vi "AlliGator Plot Fit Parameter vs Intensity v2.vi"(6 "Fit Parameter":T1, 7 "Lifetime Graph refnum":refnum<vi>, 8 "error in (no error)":errorcluster, 9 "ROI idx (2147483647: all ROIs)":i32=-1, 11 "Data Value Reference in":refnum<data-value>) -> (0 "error out":errorcluster, 3 "Data Value Reference out":refnum<data-value>)   [LabVIEW 2021, in "AlliGator Decay Fit Parameter Map.lvlib"]
doc: "Creates scatter plot of selected parameter vs intensity for all ROIs and sends it to the <B>Lifetime & Other Parameters Graph</B>."
uses:
  AlliGator Decay Fit Parameter Map.lvlib
  AlliGator Internal Variables v2.ctl
  <vilib>/vision/Image Controls.llb/IMAQ Image.ctl
  AlliGator Gate Image Set.ctl
  AlliGator FLI Dataset Type.ctl
  AlliGator Data Series Type.ctl
  AlliGator Dataset Channel.ctl
  AlliGator Gate Arithmetic.ctl
  AlliGator Displayed Image.ctl
  Image/Named ROI Description.ctl
  AlliGator Decay Metadata v3.ctl
  AlliGator Decay Background Subtraction Info.ctl
  AlliGator Baseline Subtraction Method.ctl
  Graphs/XY Graph/XY Graph Plot Shift Parameters.ctl
  Graphs/XY Graph/XY Graph Plot Shift Method.ctl
  AlliGator Decay Extrapolation Parameters.ctl
  Phasor/Calibration Phasor (m, phi).ctl
  Phasor/Phasor Reference Series.ctl
  Phasor/Phasor Calibration Map v2.ctl
  Phasor/Phasor (g, s).ctl
  AlliGator Raw Phasor Plot Data v4.ctl
  Phasor/Phasor Standard Deviation Options.ctl
  AlliGator Phasor Multi-Harmonic Data.ctl
  Phasor/Phasor Harmonic Data.ctl
  AlliGator Decay Fit Options & Parameters v2.ctl
  Fits/IRF(X)PSED/Decay Fit Options v2.ctl
  Fits/Decay Convolution/Decay Model.ctl
  Fits/Residual Type.ctl
  Fits/IRF(X)PSED/Fit Weights Type.ctl
  Fits/Non-linear Fitting Method v2.ctl
  Fits/Fit Calculation Method.ctl
  Fits/Non-linear Fitting Algorithm.ctl
  AlliGator Decay Fit Parameter Constraints 2.ctl
  Fits/IRF(X)PSED/Decay Fit Parameters In List.ctl
  Fits/IRF(X)PSED/MLE Baseline Offset Type.ctl
  AlliGator Decay Preprocessing Parameters.ctl
  Fits/IRF(X)PSED/Decay Fit Parameters & Derived Quantities List.ctl
  AlliGator Variables List.ctl
  Graphs/LabVIEW Plot Interpolation.ctl
  Graphs/Plot Point Style.ctl
  Variant/Variant to Data/Variant to U16.vi
  AlliGator Files.lvlib
  Graphs/XY Graph/XY Graph Add-Ons.lvlib
  AlliGator Globals, Variables & Constants.lvlib
  Image/Image.lvlib
  Notebook/Notebook.lvlib
  Rich Text Box/Rich Text Box.lvlib
  Variant/Variant to Data/Variant to Data.lvlib
  <vilib>/vision/NI_Vision_Development_Module.lvlib
  Graphs/Graphs.lvlib
  Phasor/Phasor.lvlib
  AlliGator Decay Preprocessing.lvlib
  AlliGator Phasor Graph.lvlib
  AlliGator Phasor Plot.lvlib
  AlliGator Source Image.lvlib
  Fits/Fits.lvlib
  AlliGator Internal Variables.lvlib
  AlliGator Decay Fit.lvlib
  AlliGator Settings.lvlib
  AlliGator Dual-Channel Datasets.lvlib
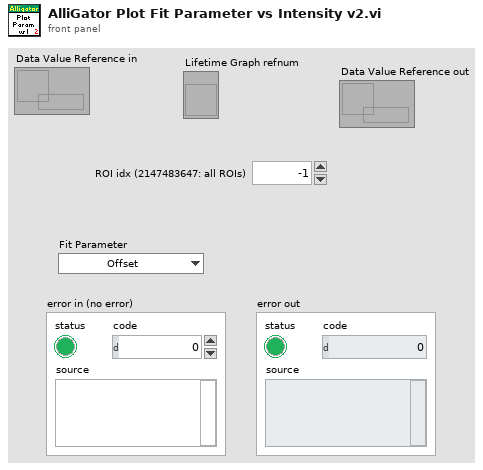
[diagram p1: front panel]
types:
  T1 = typedef "Fits.lvlib/Decay Fit Parameters & Derived Quantities List.ctl" = enum16{"Offset", "Baseline", "A_1", "tau_1", "A_2", "tau_2", "<tau>_a", "f1_a", "f2_a", "<tau>_i", "f1_i", "f2_i", "-", "R^2", "Chi^2"}
  T2 = typedef "AlliGator Globals, Variables & Constants.lvlib/AlliGator Variables List.ctl" = enum16{"---- GUI ----", "Initialization Status", "State Indicators Refnum", "Original AlliGator Menu Items", "Current Action Loop State", "Script in progress", "Playback", "Loop Playback", "Search ROI Used", "Search ROI", "Decay Graph Max Legend Size", "Intensity Graph Max Legend Size", "Decay Statistics Graph Max Legend Size", "Phasor Graph Max Legend Size", "Phasor Ratio Graph Max Legend Size", "Lifetime Graph Max Legend Size", "---- Files ----", "Export Dataset Frames as Individual Files", "Show Batch Export Help Balloons", "Frames in Dataset", "ptu File Frame Start Indices", "Current Frame in Dataset", "Current Frame Timestamp", "------ Python Plugins ------", "Python Plugins Information", "Python Session", "Valid Python Session?", "---- Source Image ----", "Dataset Loaded", "Dataset Metadata", "Dataset Channel", "Dataset Data Description", "Background Dataset Metadata", "Background Dataset Channel", "Background Dataset Data Description", "Background File Subtraction", "Background File Path", "Background File Pile-up Correction", "Background File Pixel Well Capacity", "Background File Scaling Factor", "Source Image ROIs", "Current Source Image ROI", "Source Image ROI Event Refnum", "X_Source Image Display Range", "X_Source Image Palette Information", "Source Image Palette List", "Source Image Scale", "Current Dataset Load Settings", "Source Image:ROI Overlay Color", "---- Image Profile Window ----", "Image Profile:Overlay ROI in Source Image", "Image Profile Window Event Refnum", "Image Profile:IntensityType", "Image Profile:Intensity Average Type", "Image Profile:Intensity-weighted SDV", "Image Profile:Box Profile Type", "Image Profile Window Open", "Image Profile:Plotted Fit Parameter", "X_Type of Displayed Image", "X_Time Gate Slider", "Dataset Path", "Source Image Overlay to Erase", "Is Displayed Image Accumulated", "White Light Image Modified", "Mask Image Modified", "Macrotime Gate Separation", "------ Phasor Graph -------", "Phasor Graph:Show Line", "---- Phasor Plot ---", "Phasor Plot Parameters Changed", "FLI Dataset Modified since last Phasor Plot Calculation", "Phasor Harmonics Data", "Selected Phasor Harmonics", "Phasor Harmonic Manager Event Refnum", "Phasor Plot ROIs", "Current Phasor Plot ROI", "Phasor Plot ROI Event Refnum", "Phasor Plot Image Reference Points", "Phasor Plot Computed", "Phasor Plot Palette Information", "Phasor Plot Palette List", "Phasor Ratio Palette Information", "Phasor Ratio Palette List", "Phasor Image Scale", "Phasor Plot Image Overlay to Erase", "Phasor Plot Image Elements to Update", "Current Phasor Plot Calculation Parameters", "Current Phasor Calibration Options", "Reset Cumulated Phasor Plot", "Phasor Ratio Reference 1", "Phasor Ratio Lifetime Reference 1", "Phasor Ratio Reference 1 Frequency", "Phasor Ratio Reference 2", "Phasor Ratio Lifetime Reference 2", "Phasor Ratio Reference 2 Frequency", "---- Decay Analysis ----", "Number of Selected Decays to Fit", "LS Fit Results", "LAR Fit Results", "BS Fit Results", "Last Decay Max - Min", "Best Fit Parameters", "Best Fit Parameter Names", "Actual Size X", "Actual Size Y", "Binning X", "Binning Y", "Actual # Gates", "Dataset Number", "Gates to...", "Gates Skipped", "Gates to keep", "Gate Step", "Gate Separation", "Reversed Gates", "Pile-up Correction", "Pixel Well Capacity", "Background Subtracted", "Background Subtraction Method", "Background Definition Range", "Background File (deprecated)", "Number of Dataset Accumulated", "Array of Accumulated Dataset Paths", "Do Averaged Datasets", "Destination File Path", "Process Plot Target", "Use 1/D as Phasor Frequency", "---- Decay Fit Parameter Map -----", "Decay Fit Parameter Map Palette Information", "Decay Fit Parameter Map Palette List", "Local Decay Graph Window Event Refnum", "------- Local Decay Window ---------", "Use normalized IRF for convolution", "----- Miscellaneous ----", "Skippable Dialog Windows Status"}
  T3 = typedef "Graphs.lvlib/Plot Point Style.ctl" = enum16{"not defined", "None", "Empty Circle", "Filled Circle", "Thick Circle", "Dotted Circle", "Empty Square", "Filled Square", "Thick Square", "Dotted Square", "Small Filled Square", "Dot", "Cross", "Tiny Cross", "Large X", "Small x", "Diamond", "Small Empty Square"}
  T4 = typedef "Image.lvlib/Named ROI Description.ctl" = cluster{"ROI Descriptor":T5, "ROI Name":string, "Overlay Color":u32}
  T5 = typedef "ROI Descriptor" = cluster{"Global Rectangle":i32[], "Contours":cluster{"ID":enum32{"External", "Internal"}, "Type":u32, "Coordinates":i32[]}[]}
  T6 = typedef "AlliGator Internal Variables.lvlib/AlliGator Internal Variables v2.ctl" = cluster{"Displayed Image":T7, "White Light Image":T7, "Mask Image":T7, "ROI Mask Image":T7, "Current Dataset Images 1":T8, "Background Dataset Images 1":T8, "Current Dataset Images 2":T8, "Background Dataset Images 2":T8, "Current Dataset Arithmetic Images":T8, "Accumulated Dataset Images 1":T8, "Accumulated Dataset Images 2":T8, "Accumulated Dataset Arithmetic Images":T8, "Phasor Plot Image":T7, "Decay Fit Parameter Map Image":T7, "Single Data Point Path":path, "White Light Image Path":path, "Mask Image Path":path, "Time-Series Folder":path, "[Time-Series Paths]":path[], "Current Dataset":i32, "Single Dataset Type":T9, "Current Folder":string, "AlliGator Data Series Type":T10, "# Datasets":i32, "Dual-Channel Dataset":bool, "Selected Channel Name":string, "Dataset Channel":T11, "Channel Arithmetic":T12, "Dual-Channel Background Dataset":bool, "Background Channel":T11, "Dual-Channel Accumulated Dataset":bool, "Start Time":dbl, "[Time-Series Timestamps]":dbl[], "[Intensity Corrections]":dbl[], "Time Series Script":bool, "Type of Displayed Image":T13, "Gate Image Slide":u16, "# Gates":i32, "ROIs":T4[], "ROI Decay":cluster{"t Array":dbl[], "I Array":dbl[]}, "Valid Decay":bool, "Decay  Metadata":T14, "Reference Decay Plot Name":string, "Reference Decay":cluster{"t Array":dbl[], "I Array":dbl[]}, "Decay Shift Plot":cluster{"Time Stamps":dbl[], "Decay Shifts":dbl[]}, "[Decays Max Values]":sgl[], "[Decays Min Values]":sgl[], "Calibration Phasor":T20, "Calibration Phasor Series":T21, "Phasor Calibration Map":T22, "Calibration Map MD5 Digest":string, "Last Raw Phasor":T23, "Last Calibrated Phasor":T23, "Last Calibrated Phasor SDV":T23, "Phasor Graph:Phasor Plot":cluster{"g Array":dbl[], "s Array":dbl[]}, "Phasor Graph:Phasor SDV Plot":cluster{"g Array":dbl[], "s Array":dbl[]}, "[Phasor Graph:Raw Phasor Plots]":T24[], "Phasor Plot locked to Ref 1":i32, "[Phasor Plot(s) locked to Ref 1]":i32[], "[Phasor Plot(s) locked to Ref 2]":i32[], "[Pixel Phasors]":T23[], "[[Sum Image]]":dbl[][], "[[CSG Phasors]]":csg[][], "[[Valid Pixel?]]":bool[][], "I/m/phi Dataset":cluster{"I/m/phi Dataset?":bool, "Base Frequency":dbl[unit], "Harmonic Orders":u8[]}, "Multi Phasor Plot Data":T26, "Decay Fit Options & Parameters":T28, "Fit Options: Decay Preprocessing Parameters":T39, "Fit Options: Reference Decay":cluster{"t Array":dbl[], "I Array":dbl[]}, "Is Full Image Parameters Map":bool, "Is Single-Pixels Parameters Map":bool, "NLSF Parameters Map X Resolution":i32, "NLSF Parameters Map Y Resolution":i32, "[Single Decay Fit Parameters]":dbl[], "Fit Model":T30, "[[Multiple Decays Fit Parameters]]":dbl[][], "[[Multiple Decays Fit Parameter SDVs]]":dbl[][], "[[IRFs]]":dbl[][], "IRF Array Time Axis":dbl[], "Decay Array Time Axis":dbl[], "[Decay Fit Parameter Names]":T1[], "[[Phasor Ratios]]":dbl[][], "[[Average Lifetimes]]":dbl[][], "Amplitude Weighted Average Lifetime":bool, "[Decay Sum]":dbl[], "[[User-defined Quantities]]":dbl[][], "User-defined Quantity":string}
  T7 = typedef "IMAQ Image.ctl" = refnum<image>
  T8 = typedef "AlliGator Files.lvlib/AlliGator Gate Image Set.ctl" = cluster{"SGL Image Max":T7, "SGL Image Sum":T7, "SGL Gate Images":T7[], "SGL Image Min":T7}
  T9 = typedef "AlliGator Files.lvlib/AlliGator FLI Dataset Type.ctl" = enum16{"HDF5 FLI Dataset", "Gate Image Folder", ".sdt FLI Dataset (Becker & Hickl)", ".ptu FLI Dataset (PicoQuant)", "SS1 FLI Dataset", "SS2 FLI Dataset", "I/m/phi Dataset", ".bin FLI Dataset (PicoQuant Binned)", ".bin FLI Dataset (Piccolo Binned)"}
  T10 = typedef "AlliGator Files.lvlib/AlliGator Data Series Type.ctl" = enum16{"Not a Supported Series", "Gate Images Folder Series", "SwissSPAD 2 Dataset Series", "B&H FLI Dataset Series", "PicoQuant PTU FLI Dataset Series", "PicoQuant BIN FLI Dataset Series", "Piccolo hist BIN FLI Dataset Series", "HDF5 FLI Dataset Series"}
  T11 = typedef "AlliGator Dual-Channel Datasets.lvlib/AlliGator Dataset Channel.ctl" = enum16{"G2", "INT"}
  T12 = typedef "AlliGator Settings.lvlib/AlliGator Gate Arithmetic.ctl" = enum16{"None", "INT-G2", "G2/INT*<INT>", "(1 - G2/INT)*<INT>"}
  T13 = typedef "AlliGator Source Image.lvlib/AlliGator Displayed Image.ctl" = enum16{"Single Gate", "Sum of All Gates", "Max of All Gates", "Min of All Gates", "-", "White Ligth Image", "Mask Image"}
  T14 = typedef "AlliGator Phasor Graph.lvlib/AlliGator Decay Metadata v3.ctl" = cluster{"ROI Descriptor":T5, "ROI Center":cluster{"X":i32, "Y":i32}, "Decay Background Subtraction Info":T15, "Decay Reverted":bool, "Decay Smoothened":bool, "Decay Straightened":bool, "Fitted Tau (Decay Straightening)":dbl, "Decay Shift Parameters":T17, "Decay Shifted":bool, "Decay Extrapolated":bool, "Decay Extrapolation Parameters":T19, "Decay Normalized":bool, "Fold Decay":bool, "# Folds":u32}
  T15 = typedef "AlliGator Decay Analysis.lvlib/AlliGator Decay Preprocessing.lvlib/AlliGator Decay Background Subtraction Info.ctl" = cluster{"Laser Period":dbl[unit], "Gate Duration":dbl[unit], "Baseline Subtraction Method":T16, "Background Definition Range":cluster{"Min Gate":dbl[unit], "Max Gate":dbl[unit]}, "Total Intensity w/o Bkgd Subtraction":dbl, "Bkgd-subtracted Intensity (exp)":dbl, "# Data Points":i32, "Background/Gate":dbl, "Fitted Lifetime":dbl[unit], "Bkgd-subtracted Intensity (theo)":dbl}
  T16 = typedef "AlliGator Decay Analysis.lvlib/AlliGator Decay Preprocessing.lvlib/AlliGator Baseline Subtraction Method.ctl" = enum16{"Mean", "Min", "Square Gated Single-Exponential", "File", "Constant"}
  T17 = typedef "XY Graph Add-Ons.lvlib/XY Graph Plot Shift Parameters.ctl" = cluster{"Type":T18, "Shift":dbl[unit], "Threshold":dbl, "Rotate":bool}
  T18 = typedef "XY Graph Add-Ons.lvlib/XY Graph Plot Shift Method.ctl" = enum16{"Default", "CFD", "Threshold", "Cross-Correlation"}
  T19 = typedef "AlliGator Decay Analysis.lvlib/AlliGator Decay Preprocessing.lvlib/AlliGator Decay Extrapolation Parameters.ctl" = cluster{"Additional Points":u32, "Head Fraction":dbl, "Fitted Tau":dbl, "Use Periodicity":bool, "Use Cursors":bool, "Tail Fraction":dbl}
  T20 = typedef "Phasor.lvlib/Calibration Phasor (m, phi).ctl" = cluster{"m":dbl, "phi":dbl, "Phasor Frequency":dbl[unit], "Reference Lifetime":dbl[unit]}
  T21 = typedef "Phasor.lvlib/Phasor Reference Series.ctl" = cluster{"m Array":dbl[], "phi Array":dbl[], "Phasor Frequency":dbl[unit], "Calibration Lifetime":dbl[unit]}
  T22 = typedef "Phasor.lvlib/Phasor Calibration Map v2.ctl" = cluster{"Phasor Frequency":dbl[unit], "Calibration Lifetime":dbl[unit], "ROI Centers":cluster{"X":i32, "Y":i32}[], "ROI Descriptors":T5[], "Map Resolution X":i32, "Map Resolution Y":i32, "z Array":cdb[]}
  T23 = typedef "Phasor.lvlib/Phasor (g, s).ctl" = cluster{"g":dbl, "s":dbl}
  T24 = typedef "AlliGator Phasor Graph.lvlib/AlliGator Raw Phasor Plot Data v4.ctl" = cluster{"Phasor Plot Name":string, "Raw Phasor Plot":T23[], "Phasor Frequency":dbl[unit], "[Decay Metadata]":T14[], "Raw Phasor Plot SDV":T23[], "Phasor SDV Options":T25, "[Calibration Phasor]":T20[]}
  T25 = typedef "Phasor.lvlib/Phasor Standard Deviation Options.ctl" = cluster{"Compute Estimated SDV":bool, "# Replicas":u32, "Use Estimated Average Phasor":bool}
  T26 = typedef "AlliGator Phasor Plot.lvlib/AlliGator Phasor Multi-Harmonic Data.ctl" = cluster{"Base Frequency":dbl[unit], "# Harmonics":u8, "Harmonic Orders":u8[], "Phasor Plot Settings Checksum":u64, "Phasor Harmonic Data Array":T27[]}
  T27 = typedef "Phasor.lvlib/Phasor Harmonic Data.ctl" = cluster{"Phasor Harmonic Name":string, "Phasor Plot Settings Checksum":u64, "Phasor Frequency":dbl[unit], "Base Frequency":dbl[unit], "Harmonic Order":u8, "Phasor Plot Parameters":string, "Phasor Array [[CSG]]":csg[][], "Dataset File Path":path}
  T28 = typedef "AlliGator Decay Fit Parameter Map.lvlib/AlliGator Decay Fit Options & Parameters v2.ctl" = cluster{"SYNC Period":dbl[unit], "Fit Options":T29, "Fit Parameter Constraints":T36[], "MLE Baseline Offset":dbl, "MLE Baseline Offset Type":T38}
  T29 = typedef "Fits.lvlib/Decay Fit Options v2.ctl" = cluster{"Show Fit Residuals":bool, "Fit Model":T30, "Residual Type":T31, "Max Decay Percentile":dbl, "Min Decay Percentile":dbl, "Show Full Decay":bool, "Weights":T32, "Fitting Method":T33, "Compute Parameter Uncertainties":bool, "Periodic Boundaries":bool, "Model Calculation":T34, "Period":dbl[unit], "Termination Criteria":cluster{"Max Iterations":i32, "Max Function Calls":i32, "Max Time":dbl[unit], "Function Tolerance":dbl, "Parameter Tolerance":dbl, "Gradient Tolerance":dbl, "Min Lambda":dbl, "Max Lambda":dbl, "Initial Tick Count":u32}, "Offset Resolution":dbl[unit], "Use Local IRF":bool, "Fitting Algorithm":T35}
  T30 = typedef "Fits.lvlib/Decay Model.ctl" = enum16{"1-Exponential", "2-Exponentials"}
  T31 = typedef "Fits.lvlib/Residual Type.ctl" = enum16{"Standard", "Normalized", "Reduced"}
  T32 = typedef "Fits.lvlib/Fit Weights Type.ctl" = enum16{"Unweighted", "1/Variance", "Best of All"}
  T33 = typedef "Fits.lvlib/Non-linear Fitting Method v2.ctl" = enum16{"Least Square", "Least Absolute Residual", "Bisquare", "MLE", "-", "Best of All"}
  T34 = typedef "Fits.lvlib/Fit Calculation Method.ctl" = enum16{"Simulation", "Convolution", "Integration"}
  T35 = typedef "Fits.lvlib/Non-linear Fitting Algorithm.ctl" = enum16{"Levenberg-Marquardt", "Trust-Region Dogleg"}
  T36 = typedef "AlliGator Decay Analysis.lvlib/AlliGator Decay Fit.lvlib/AlliGator Decay Fit Parameter Constraints 2.ctl" = cluster{"Fit Parameter":T37, "Min Value":dbl, "Max Value":dbl, "Global":bool, "Used":bool}
  T37 = typedef "Fits.lvlib/Decay Fit Parameters In List.ctl" = enum16{"Offset", "Baseline", "A_1", "tau_1", "A_2", "tau_2"}
  T38 = typedef "Fits.lvlib/MLE Baseline Offset Type.ctl" = enum32{"Absolute", "Percentage"}
  T39 = typedef "AlliGator Decay Analysis.lvlib/AlliGator Decay Preprocessing.lvlib/AlliGator Decay Preprocessing Parameters.ctl" = cluster{"Background Subtraction":bool, "Straighten Decay":bool, "Reverse Gates":bool, "1-Normalized Decay":bool, "Smoothen Decay":bool, "Smoothing Parameter":dbl, "Shift Decay":bool, "Decay Shift Parameters":T17, "Extrapolate Decay":bool, "Additional Points":u32, "Head Fraction":dbl, "Pixel-Normalize Decay":bool, "Use Periodicity":bool, "Use Cursors":bool, "Tail Fraction":dbl, "Use Decay Pre-Processing":bool, "Fold Decay":bool, "# Folds":u32, "[0-1]-Normalized Decay":bool}
  T40 = typedef "Graphs.lvlib/LabVIEW Plot Interpolation.ctl" = u8
  T41 = typedef "XY Graph Add-Ons.lvlib/XY Graph Refnum.ctl" = refnum<vi>
  T42 = typedef "Rich Text Box.lvlib/Text Formatting.ctl" = cluster{"Font":string, "Text Color":T43, "Text Background Color":T43, "Text Style":enum16{"Regular", "Bold", "Italic", "Underline", "Strikeout"}, "Font Size (Points)":dbl, "Text Alignment":i32}
  T43 = typedef "Rich Text Box.lvlib/Text Colors.ctl" = enum16{"Unchanged", "Black", "Blue", "Brown", "Gray", "Green", "Orange", "Pink", "Red", "White"}
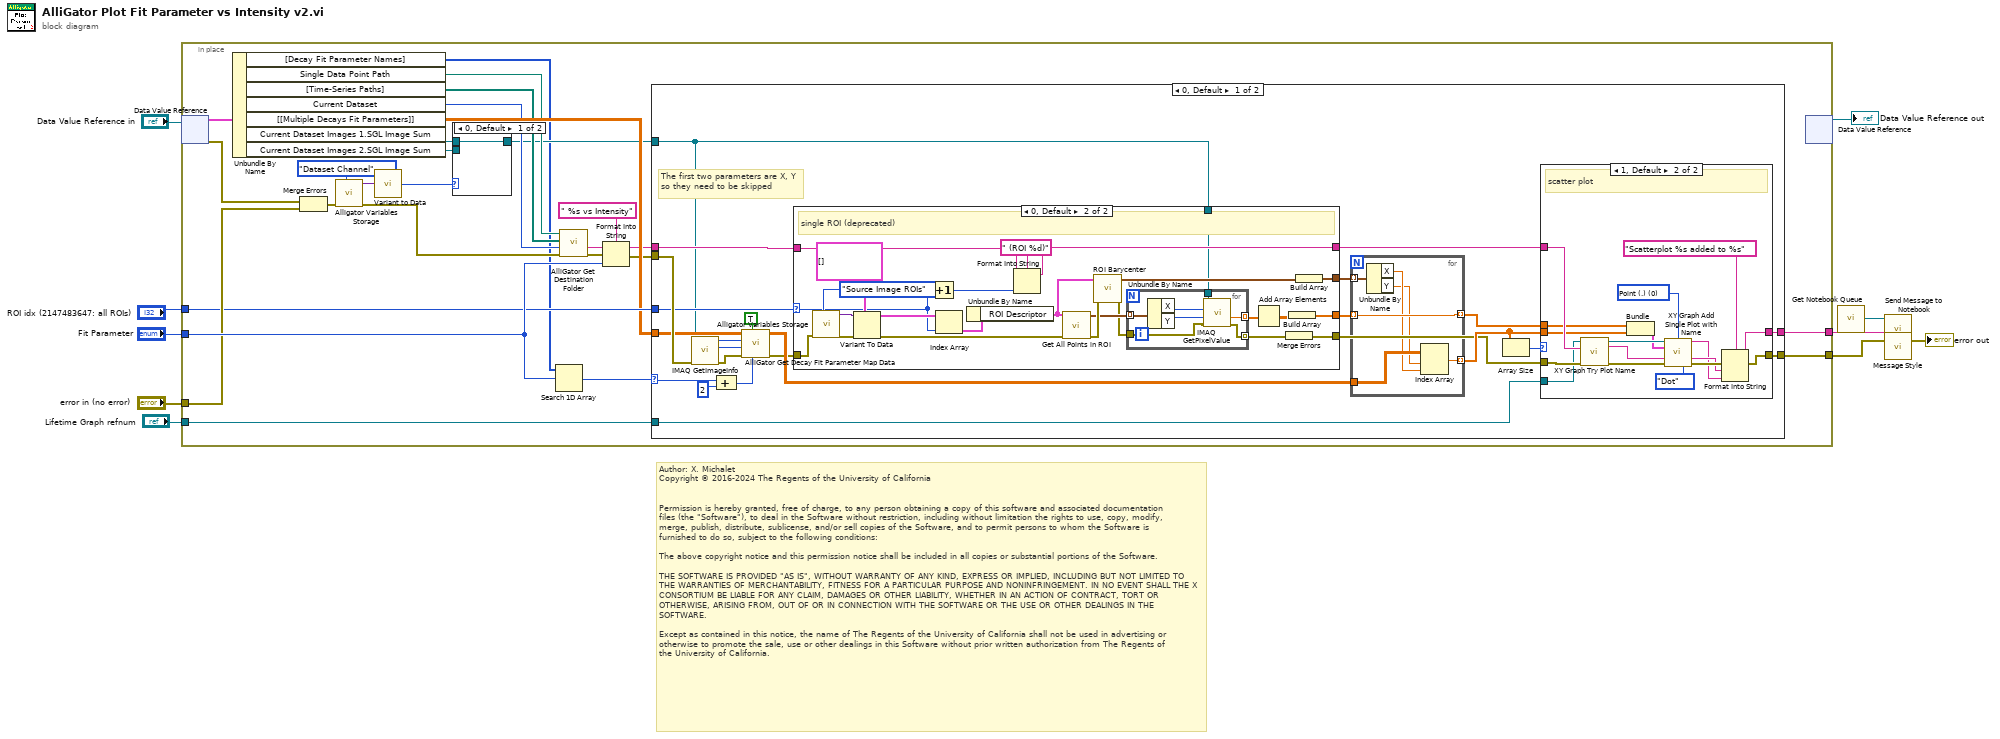
[diagram p0: block diagram]
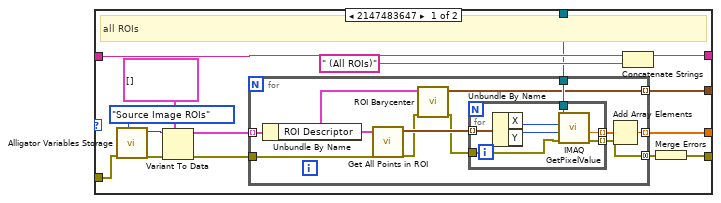
[diagram p4: hidden frame]
diagram:
  # "Author: X. Michalet\nCopyright © 2016-2024 The Regents of the University of California\n \n\nPermission is hereby granted, free of charge, to any person obtaining a copy of this software and associated documentation files (the \"Software\"), to deal in the Software without restriction, including without limitation the rights to use, copy, modify, merge, publish, distribute, sublicense, and/or sell copies of the Software, and to permit persons to whom the Software is furnished to do so, subject to the following conditions:\n\nThe above copyright notice and this permission notice shall be included in all copies or substantial portions of the Software.\n\nTHE SOFTWARE IS PROVIDED \"AS IS\", WITHOUT WARRANTY OF ANY KIND, EXPRESS OR IMPLIED, INCLUDING BUT NOT LIMITED TO THE WARRANTIES OF MERCHANTABILITY, FITNESS FOR A PARTICULAR PURPOSE AND NONINFRINGEMENT. IN NO EVENT SHALL THE X CONSORTIUM BE LIABLE FOR ANY CLAIM, DAMAGES OR OTHER LIABILITY, WHETHER IN AN ACTION OF CONTRACT, TORT OR OTHERWISE, ARISING FROM, OUT OF OR IN CONNECTION WITH THE SOFTWARE OR THE USE OR OTHER DEALINGS IN THE SOFTWARE.\n\nExcept as contained in this notice, the name of The Regents of the University of California shall not be used in advertising or otherwise to promote the sale, use or other dealings in this Software without prior written authorization from The Regents of the University of California."
  n1 = in-place {
    in-place-border: "Fit Parameter" -> [w37]
    in-place-border: "error in (no error)" -> [w36]
    in-place-border: [w34] -> w2
    in-place-border: "Lifetime Graph refnum" -> [w33]
    in-place-border: "ROI idx (2147483647: all ROIs)" -> [w32]
    in-place-border: [w31] -> w3
    n2 = in-place-dvr #1("Data Value Reference in") -> (w38:T6, w35:errorcluster)
    n3 = Unbundle By Name(w38) -> ("[Decay Fit Parameter Names]"=w12:T1[], "Single Data Point Path"=w26:path, "[Time-Series Paths]"=w25:path[], "Current Dataset"=w24:i32, "[[Multiple Decays Fit Parameters]]"=w27:dbl[][], "Current Dataset Images 1.SGL Image Sum"=w22:T7, "Current Dataset Images 2.SGL Image Sum"=w16:T7)
    n4 = Merge Errors(w35, w36) -> (w18:errorcluster)
    n5 = call "Alligator Variables Storage.vi"("AlliGator Variable"=AlliGator_Variables_List."Dataset Channel" ("Alligator Variable"), "Error In"=w18) -> ("Error Out"=w14:errorcluster, "Data out"=w19:variant)  [unwired: 7 in, 1 out]
    n6 = call-poly "Variant to Data.vi"("Variant"=w19) -> ("U16 Value"=w17:u16)  [unwired: 8 in]
    n7 = case shown="0, Default" w17 {
      tunnel: [w39 w40] -> w21
      tunnel: w16 -> [_ w40]
      tunnel: w22 -> [w39 _]
      frame 0, Default {
      }
      frame 1 {
      }
    }
    n8 = Search 1D Array(1D array=w12, element=w37) -> (index of element=w28:i32)  [unwired: 1 in]
    n9 = call "AlliGator Get Destination Folder.vi"("Error In"=w14, "Current Data Set (-1: single)"=w24, "Time-Series Paths"=w25, "Single Data Point Path"=w26) -> ("Error Out"=w15:errorcluster, "Data Point Name"=w30:string)  [unwired: 5 in, 1 out]
    n10 = Format Into String(format string=" %s vs Intensity", initial string=w30, error in=w15, w37) -> (resulting string=w23:string, error out=w13:errorcluster)
    n11 = case shown="0, Default" w28 {
      selector: w28 -> [w62 _]
      tunnel: w13 -> [w63 w154]
      tunnel: w21 -> [w44 _]
      tunnel: w27 -> [w51 _]
      tunnel: [w60 w154] -> w34
      tunnel: w23 -> [w55 _]
      tunnel: w33 -> [w45 _]
      tunnel: w32 -> [w59 _]
      tunnel: [w53 _] -> w31
      frame 0, Default {
        # "The first two parameters are X, Y so they need to be skipped"
        n12 = call "IMAQ GetImageInfo"("error in (no error)"=w63, "Image"=w44) -> ("error out"=w48:errorcluster, "Y Resolution"=w49:i32, "X Resolution"=w50:i32)  [unwired: 2 in, 5 out]
        n13 = Compound Arithmetic op=ADD(w62, 2 ("value")) -> (w64:i32)
        n14 = call "AlliGator Get Decay Fit Parameter Map Data.vi"("Map index"=w64, "Compute Decay Fit Parameter Map"=TRUE, "Error In"=w48, "Y Resolution"=w49, "X Resolution"=w50, "Multiple Decays Fit Parameters"=w51) -> ("Error Out"=w58:errorcluster, "Map Data (V x H)"=w61:dbl[][])  [unwired: 3 in, 1 out]
        n15 = case shown="0, Default" w59 {
          selector: w59 -> [_ w136]
          tunnel: [w92 w126] -> w41
          tunnel: w58 -> [w98 w142]
          tunnel: w55 -> [w97 w140]
          tunnel: [w96 w138] -> w54
          tunnel: w44 -> [w91 w124]
          tunnel: [w90 w122] -> w43
          tunnel: [w89 w133] -> w42
          frame 2147483647 {
            # "all ROIs"
            n16 = call "Alligator Variables Storage.vi"("AlliGator Variable"=AlliGator_Variables_List."Source Image ROIs" ("Alligator Variable"), "Error In"=w98) -> ("Error Out"=w101:errorcluster, "Data out"=w102:variant)  [unwired: 7 in, 1 out]
            n17 = Variant To Data(error in=w101, type=T4[] [] ("ROIs"), Variant=w102) -> (data=w99:T4[], error out=w94:errorcluster)
            n18 = for {
              tunnel: w99 -> [w114] mode=indexing
              tunnel: w94 -> [w113]
              tunnel: [w104] -> w93 mode=concatenating
              tunnel: w91 -> [w111]
              tunnel: [w109] -> w90 mode=indexing
              tunnel: [w106] -> w89 mode=indexing
              n19 = Unbundle By Name(w114) -> ("ROI Descriptor"=w108:T5)
              n20 = call "Get All Points in ROI.vi"("Error In"=w113, "ROI Descriptor"=w108) -> ("Error Out"=w107:errorcluster, "Point Array"=w112:cluster{"X":i32, "Y":i32}[])  [unwired: 8 in]
              n21 = call "ROI Barycenter.vi"("Error In"=w107, "ROI Descriptor in"=w108) -> ("Error Out"=w105:errorcluster, "ROI Center"=w106:cluster{"X":dbl, "Y":dbl})  [unwired: 8 in]
              n22 = for {
                tunnel: w112 -> [w121] mode=indexing
                tunnel: w111 -> [w118]
                tunnel: [w117] -> w110 mode=indexing
                tunnel: w105 -> [w116]
                tunnel: [w115] -> w104 mode=indexing
                n23 = Unbundle By Name(w121) -> ("X"=w120:i32, "Y"=w119:i32)
                n24 = call "IMAQ GetPixelValue"("Image"=w118, "X Coordinate"=w120, "Y Coordinate"=w119, "error in (no error)"=w116) -> ("Pixel Value (Float)"=w117:sgl, "error out"=w115:errorcluster)  [unwired: 2 in, 3 out]
              }
              n25 = Add Array Elements(numeric array=w110) -> (sum=w109:sgl)
            }
            n26 = Concatenate Strings(w97, " (All ROIs)" ("string")) -> (w96:string)
            n27 = Merge Errors(w93) -> (w92:errorcluster)
          }
          frame 0, Default {
            # "single ROI (deprecated)"
            n28 = call "Alligator Variables Storage.vi"("AlliGator Variable"=AlliGator_Variables_List."Source Image ROIs" ("Alligator Variable"), "Error In"=w142) -> ("Error Out"=w144:errorcluster, "Data out"=w145:variant)  [unwired: 7 in, 1 out]
            n29 = Variant To Data(error in=w144, type=T4[] [] ("ROIs"), Variant=w145) -> (data=w137:T4[], error out=w131:errorcluster)
            n30 = Increment(x=w136) -> (x+1=w135:i32)
            n31 = Index Array(array=w137, index=w136) -> (element=w141:T4)
            n32 = Unbundle By Name(w141) -> ("ROI Descriptor"=w132:T5)
            n33 = Format Into String(format string=" (ROI %d)", initial string=w140, w135) -> (resulting string=w138:string)  [unwired: 1 in, 1 out]
            n34 = call "Get All Points in ROI.vi"("Error In"=w131, "ROI Descriptor"=w132) -> ("Error Out"=w130:errorcluster, "Point Array"=w129:cluster{"X":i32, "Y":i32}[])  [unwired: 8 in]
            n35 = call "ROI Barycenter.vi"("Error In"=w130, "ROI Descriptor in"=w132) -> ("Error Out"=w128:errorcluster, "ROI Center"=w134:cluster{"X":dbl, "Y":dbl})  [unwired: 8 in]
            n36 = for {
              tunnel: w129 -> [w153] mode=indexing
              tunnel: w124 -> [w147]
              tunnel: [w150] -> w125 mode=indexing
              tunnel: w128 -> [w149]
              tunnel: [w148] -> w127 mode=indexing
              n37 = Unbundle By Name(w153) -> ("X"=w152:i32, "Y"=w151:i32)
              n38 = call "IMAQ GetPixelValue"("Image"=w147, "X Coordinate"=w152, "Y Coordinate"=w151, "error in (no error)"=w149) -> ("Pixel Value (Float)"=w150:sgl, "error out"=w148:errorcluster)  [unwired: 2 in, 3 out]
            }
            n39 = Add Array Elements(numeric array=w125) -> (sum=w123:sgl)
            n40 = Merge Errors(w127) -> (w126:errorcluster)
            n41 = Build Array(w123) -> (w122:sgl[])
            n42 = Build Array(w134) -> (w133:cluster{"X":dbl, "Y":dbl}[])
          }
        }
        n43 = for {
          tunnel: w61 -> [w88]
          tunnel: [w87] -> w57 mode=indexing
          tunnel: [w86] -> w47 mode=indexing
          tunnel: w43 -> [w86] mode=indexing
          tunnel: w42 -> [w85] mode=indexing
          n44 = Unbundle By Name(w85) -> ("X"=w84:dbl, "Y"=w83:dbl)
          n45 = Index Array(array=w88, index (row)=w83, index (col)=w84) -> (element=w87:dbl)
        }
        n46 = Array Size(array=w57) -> (size(s)=w56:i32)
        n47 = case shown="1, Default" w56 {
          tunnel: w41 -> [w65 w82]
          tunnel: w54 -> [_ w81]
          tunnel: w45 -> [_ w80]
          tunnel: [w65 w75] -> w60
          tunnel: w57 -> [_ w71]
          tunnel: [_ w69] -> w53
          tunnel: w47 -> [_ w68]
          frame 0 {
            # "No data"
          }
          frame 1, Default {
            w67 = T40 0 items=["Point (.)", "Stepwise Right (--.)", "Line + Point (\\. /)", "Stepwise Left (.--)", "Stepwise Centered (-.-)", "Stepwise Vertical (|.|)", "Line (-)", "Use Previous Plot's Style"] ("Plot Interpolation (Previous Plot's Style)")
            # "scatter plot"
            n48 = call "XY Graph Try Plot Name.vi"("Error In"=w82, "Plot Name in"=w81, "XY Graph Refnum"=w80) -> ("Error Out"=w79:errorcluster, "Plot Name out"=w78:string, "XY Graph Refnum"=w77:T41)  [unwired: 5 in, 1 out]
            n49 = Bundle(w68, w71) -> (w70:cluster{sgl[], dbl[]})  [unwired: 1 in]
            n50 = call "XY Graph Add Single Plot with Name.vi"("XYGraph Ref in"=w77, "Plot Interpolation (Previous Plot's Style)"=w67, "Plot"=w70, "Plot Name (\"Plot\")"=w78, "error in (no error)"=w79, "Point Style (Dot)"=Plot_Point_Style."Dot") -> ("XY Graph Caption (or Label)"=w73:string, "Plot Name"=w74:string, "error out"=w76:errorcluster)  [unwired: 6 in, 1 out]
            n51 = Format Into String(format string="Scatterplot %s added to %s", error in=w76, w74, w73) -> (resulting string=w69:string, error out=w75:errorcluster)  [unwired: 1 in]
          }
        }
      }
      frame -1 {
      }
    }
    n52 = in-place-dvr #1() -> (→"Data Value Reference out":refnum<data-value>)  [unwired: 1 in, 1 out]
  }
  n53 = call "Get Notebook Queue.vi"() -> ("Notebook Queue"=w4:refnum<queue>)  [unwired: 9 in]
  n54 = call "Message Style.vi"() -> ("Message Formatting"=w5:T42)
  n55 = call "Send Message to Notebook.vi"("Text Formatting"=w5, "Error In"=w2, "Message"=w3, "Notebook Queue"=w4) -> ("Error Out"=→"error out":errorcluster)  [unwired: 4 in, 1 out]
